vi "Global.vi"() -> ()   [LabVIEW 2020, in "Approval Tests.lvlib"]
uses:
  Approval Tests.lvlib
  LVCompare Options.ctl
panel:
  in  "TimeOut on Error":i32=250
  in  "Retries":i32=10
  in  "compare options":T1={"VI Attributes"=TRUE, "Front Panel"=TRUE, "FP position/size"=TRUE, "Block Diagram"=TRUE, "BD cosmetic"=TRUE, "BD position/size"=TRUE}
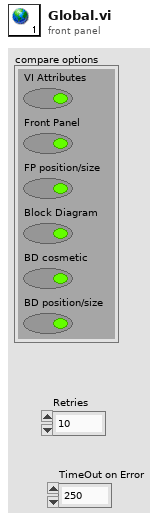
[diagram p1: front panel]
types:
  T1 = typedef "Approval Tests.lvlib/LVCompare Options.ctl" = cluster{"VI Attributes":bool, "Front Panel":bool, "FP position/size":bool, "Block Diagram":bool, "BD cosmetic":bool, "BD position/size":bool}
diagram:
